vi "Save Image.vi"(8 "error in (no error)":errorcluster, 11 "HIJ Vision Camera App In":refnum<class "HIJ Vision Camera App.lvclass">) -> (0 "error out":errorcluster, 2 "image path":path, 3 "HIJ Vision Camera App Out":refnum<class "HIJ Vision Camera App.lvclass">)   [LabVIEW 2020, in "HIJ Vision Camera App.lvlib" / "HIJ Vision Camera App.lvclass"]
doc: "Speichert das Kamerabild in PNG Format und ruft Generate Report auf. Wenn Flag \"Time in Filename\" gesetzt ist, wird ein Zeitstempel dem Dateinamen angehängt."
uses:
  HIJ Vision Camera App.lvclass
  C:/Users/AlexK/work/LabVIEW Programme/POLARIS CAM Log Abw und E/Submodules/HIJ Vision/Application Base Actors/HIJ Vision Application/HIJ Vision Application/HIJ Vision Application.lvclass
  HIJ Vision Application/HIJ Vision Application/HIJ Vision Application.lvclass/HIJ Vision Application.ctl
  HIJ Vision Camera App.lvclass/HIJ Vision Camera App.ctl
  HIJ Vision Application/HIJ Vision Application/Read Raw Image.vi
  HIJ Vision Application/HIJ Vision Application/Read WorkDir.vi
  Read Prefix.vi
  Read Camera Name.vi
  Read Save Source in Filename.vi
  Read ShotIdInFileName.vi
  HIJ Vision Application/HIJ Vision Application/Read ShotID.vi
  Read FrameNrInFilename.vi
  Read Frame Nr.vi
  Read TimestampFormat.vi
  Read ImageTimeStamp.vi
  Read SaveTimestamp.vi
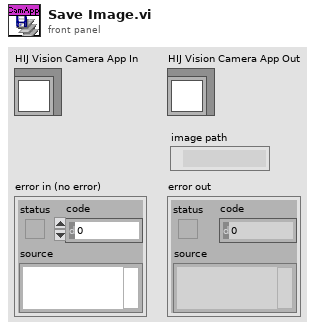
[diagram p1: front panel]
types:
  T1 = typedef "IMAQ Image.ctl" = refnum<image>
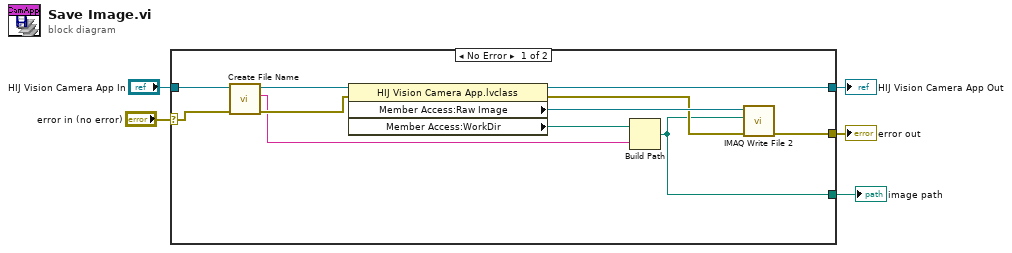
[diagram p0: block diagram]
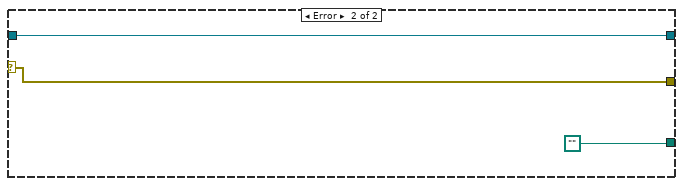
[diagram p2: hidden frame]
diagram:
  n1 = case shown="No Error" "error in (no error)" {
    selector: "error in (no error)" -> [w7 w19]
    tunnel: [w13 w19] -> w4
    tunnel: [w11 w18] -> w2
    tunnel: "HIJ Vision Camera App In" -> [w16 w18]
    tunnel: [w10 path ""] -> w1
    frame No Error {
      n2 = call-dynamic "Create File Name.vi"("error in (no error)"=w7, "HIJ Vision Camera App in"=w16) -> ("error out"=w8:errorcluster, "FileName"=w6:string, "HIJ Vision Camera App out"=w9:refnum<class "HIJ Vision Camera App.lvclass">)  [unwired: 7 in]
      n3 = property class="HIJ Vision Camera App.lvclass"(reference=w9, error in=w8) -> (reference out=w11:refnum<class "HIJ Vision Camera App.lvclass">, error out=w12:errorcluster, "Member Access:Raw Image"=w15:T1, "Member Access:WorkDir"=w14:path)
      n4 = Build Path(base path=w14, name or relative path=w6) -> (appended path=w10:path)
      n5 = call-poly "IMAQ Write File 2"("error in (no error)"=w12, "File Path"=w10, "Image"=w15) -> ("error out"=w13:errorcluster)  [unwired: 7 in, 1 out]
    }
    frame Error {
    }
  }
  "error out" <- w4
  "HIJ Vision Camera App Out" <- w2
  "image path" <- w1
